vi "Reflect Clothoid Points.vi"(9 "Rotation":dbl, 10 "Sign":cluster{"Numeric":dbl, "Numeric":dbl}, 11 "Points in":cluster{dbl, dbl}[](array[cluster])) -> (3 "Points out":cluster{dbl, dbl}[](array[cluster]))   [LabVIEW 2020]
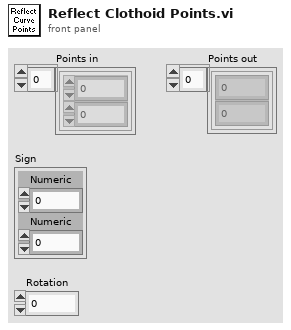
[diagram p1: front panel]
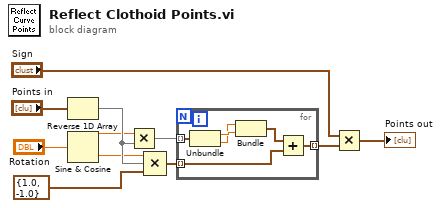
[diagram p0: block diagram]
diagram:
  n1 = Reverse 1D Array(array="Points in") -> (reversed array=w5:cluster{dbl, dbl}[])
  n2 = Sine & Cosine(0:"Rotation") -> (1:w4:dbl, 2:w3:dbl)
  n3 = Multiply(x=w4, y=w5) -> (x*y=w6:cluster{dbl, dbl}[])
  n4 = Compound Arithmetic op=MULTIPLY(w3, w5, cluster{dbl, dbl} {1.0, -1.0}) -> (w7:cluster{dbl, dbl}[])
  n5 = for {
    tunnel: w6 -> [w14] mode=indexing
    tunnel: w7 -> [w12] mode=indexing
    tunnel: [w16] -> w11 mode=indexing
    n6 = Unbundle(w14) -> (w17:dbl, w15:dbl)
    n7 = Bundle(w15, w17) -> (w13:cluster{dbl, dbl})  [unwired: 1 in]
    n8 = Add(x=w13, y=w12) -> (x+y=w16:cluster{dbl, dbl})
  }
  n9 = Multiply(x="Sign", y=w11) -> (x*y=→"Points out":cluster{dbl, dbl}[])
